vi "form_archive.vi"(0 "C7NI6703":T16, 1 "C2NI6071E 2":T10, 2 "C1NI6071E":T9, 3 "C6NI6703":T15, 5 "C1011NI6602":T14, 7 "C9NI6703":T11, 9 "C2NI6071E":T10, 12 "C5_IN_DIO96":T12, 13 "C8NI6703":T17, 14 "VAM-A":T13) -> (4 "archive out":T1)   [LabVIEW 2020]
uses:
  archive.ctl
  sync_type_def.ctl
  HT_type-def.ctl
  HF_type_def.ctl
  vacuum_type_def.ctl
  modulator_type_def.ctl
  water_cooling_type_def.ctl
  all_magnets_type_def.ctl
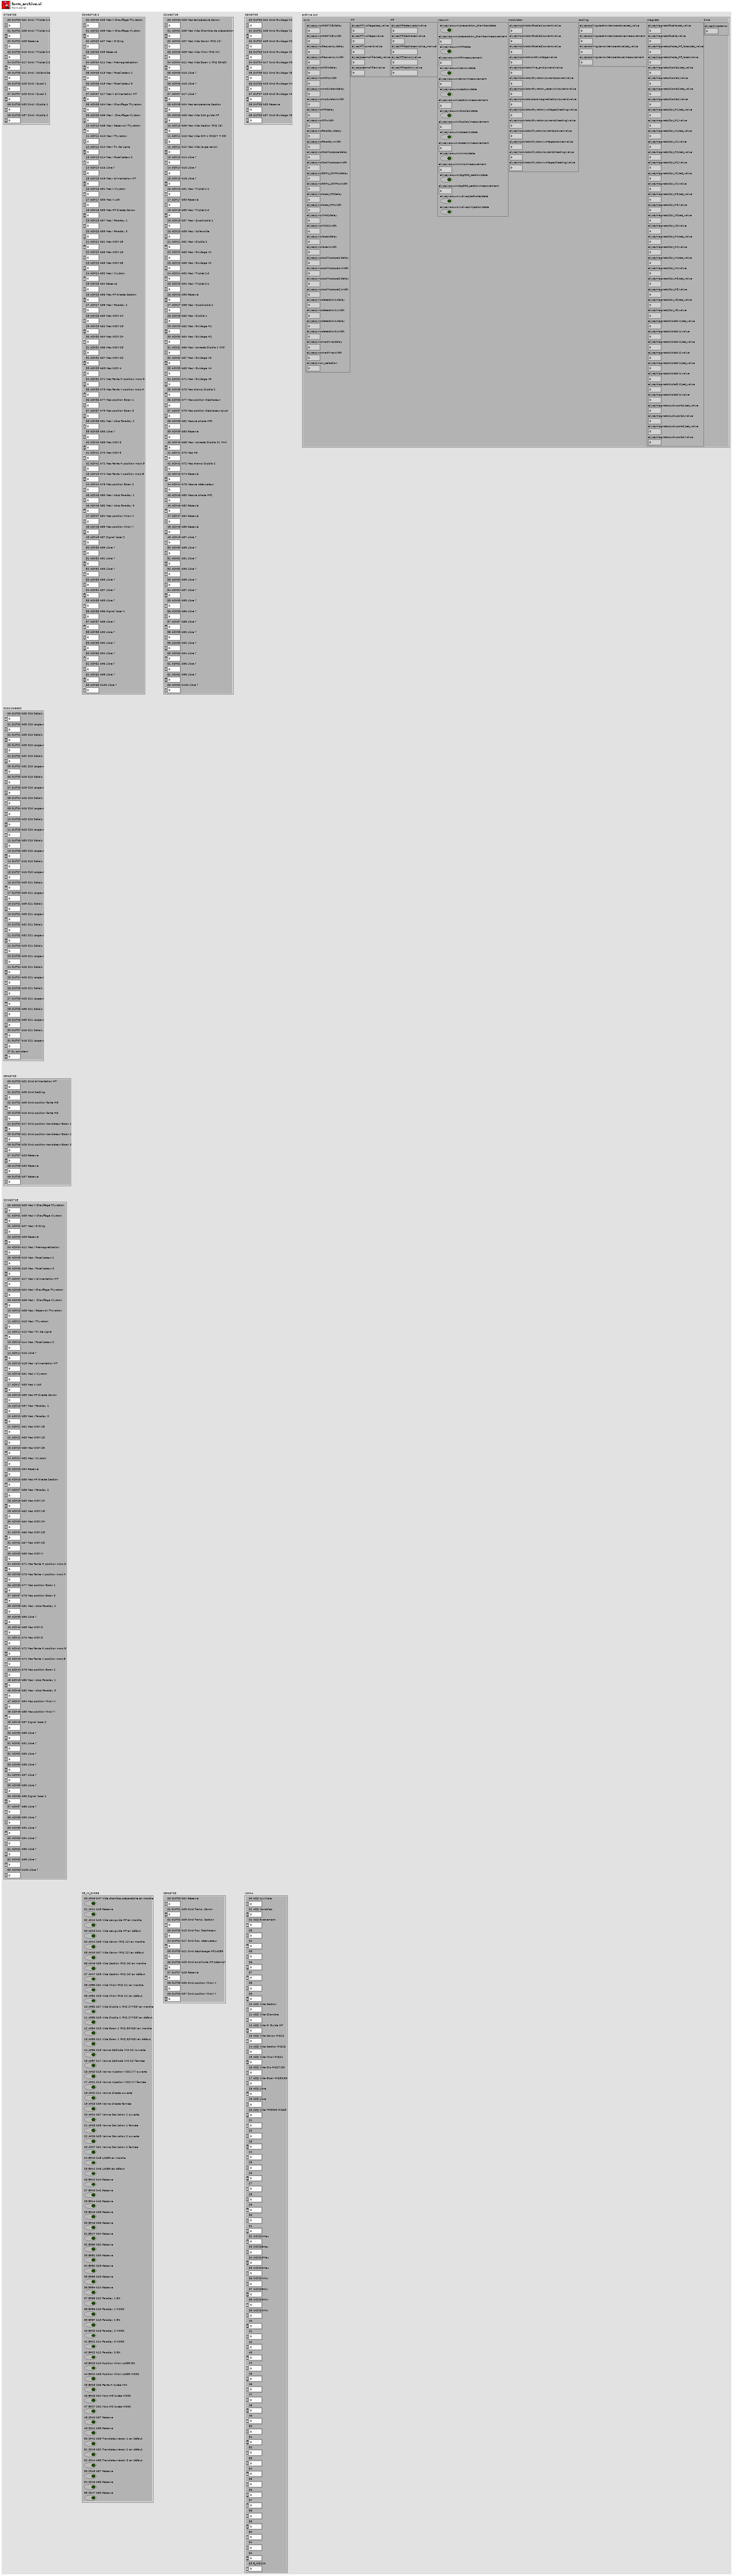
[diagram p1: front panel]
types:
  T1 = typedef "archive.ctl" = cluster{"sync":T2, "HT":T3, "HF":T4, "vacuum":T5, "modulator":T6, "cooling":T7, "magnets":T8, "time":cluster{"elyse/timestamp":dbl}}
  T2 = typedef "sync_type_def.ctl" = cluster{"elyse/sync/NI6071E/delay":dbl, "elyse/sync/NI6071E/width":dbl, "elyse/sync/frequency/delay":dbl, "elyse/sync/frequency/width":dbl, "elyse/sync/WCM/delay":dbl, "elyse/sync/WCM/width":dbl, "elyse/sync/modulator/delay":dbl, "elyse/sync/modulator/width":dbl, "elyse/sync/HF/delay":dbl, "elyse/sync/HF/width":dbl, "elyse/sync/Faraday/delay":dbl, "elyse/sync/Faraday/width":dbl, "elyse/sync/Oscilloscope/delay":dbl, "elyse/sync/Oscilloscope/width":dbl, "elyse/sync/50Hz_20MHz/delay":dbl, "elyse/sync/50Hz_20MHz/width":dbl, "elyse/sync/laser_HF/delay":dbl, "elyse/sync/laser_HF/width":dbl, "elyse/sync/IMAC/delay":dbl, "elyse/sync/IMAC/width":dbl, "elyse/sync/laser/delay":dbl, "elyse/sync/laser/width":dbl, "elyse/sync/oscilloscope1/delay":dbl, "elyse/sync/oscilloscope1/width":dbl, "elyse/sync/oscilloscope2/delay":dbl, "elyse/sync/oscilloscope2/width":dbl, "elyse/sync/detection1/delay":dbl, "elyse/sync/detection1/width":dbl, "elyse/sync/detection1/delay":dbl, "elyse/sync/detection2/width":dbl, "elyse/sync/machine/delay":dbl, "elyse/sync/machine/width":dbl, "elyse/sync/n_selection":dbl}
  T3 = typedef "HT_type-def.ctl" = cluster{"elyse/HT/voltage/set_value":dbl, "elyse/HT/voltage/value":dbl, "elyse/HT/current/value":dbl, "elyse/preamplifier/set_value":dbl, "elyse/preamplifier/value":dbl}
  T4 = typedef "HF_type_def.ctl" = cluster{"elyse/HF/attenuator/value":dbl, "elyse/HF/dephaser/value":dbl, "elyse/HF/dephaser/value_manuel":dbl, "elyse/HF/canon/value":dbl, "elyse/HF/section/value":dbl}
  T5 = typedef "vacuum_type_def.ctl" = cluster{"elyse/vacuum/preparation_chamber/state":bool, "elyse/vacuum/preparation_chamber/measurement":dbl, "elyse/vacuum/HF/state":bool, "elyse/vacuum/HF/measurement":dbl, "elyse/vacuum/canon/state":bool, "elyse/vacuum/canon/measurement":dbl, "elyse/vacuum/section/state":bool, "elyse/vacuum/section/measurement":dbl, "elyse/vacuum/dipole1/state":bool, "elyse/vacuum/dipole1/measurement":dbl, "elyse/vacuum/screen1/state":bool, "elyse/vacuum/screen1/measurement":dbl, "elyse/vacuum/mirror/state":bool, "elyse/vacuum/mirror/measurement":dbl, "elyse/vacuum/tpg300_section/state":bool, "elyse/vacuum/tpg300_section/measurement":dbl, "elyse/vacuum/valves/cathode/state":bool, "elyse/vacuum/valves/injection/state":bool}
  T6 = typedef "modulator_type_def.ctl" = cluster{"elyse/modulator/focale1/current/value":dbl, "elyse/modulator/focale2/current/value":dbl, "elyse/modulator/focale3/current/value":dbl, "elyse/modulator/LAR/voltage/value":dbl, "elyse/modulator/line_end/current/value":dbl, "elyse/modulator/thyratron/currents/power/value":dbl, "elyse/modulator/thyratron_reservoir/current/value":dbl, "elyse/modulator/paramagnetization/current/value":dbl, "elyse/modulator/thyratron/voltages/heating/value":dbl, "elyse/modulator/thyratron/currents/heating/value":dbl, "elyse/modulator/klystron/currents/power/value":dbl, "elyse/modulator/klystron/voltages/power/value":dbl, "elyse/modulator/klystron/currents/heating/value":dbl, "elyse/modulator/klystron/voltages/heating/value":dbl}
  T7 = typedef "water_cooling_type_def.ctl" = cluster{"elyse/cooling/section/temperature/set_value":dbl, "elyse/cooling/section/temperature/measurement":dbl, "elyse/cooling/canon/temperature/set_value":dbl, "elyse/cooling/canon/temperature/measurement":dbl}
  T8 = typedef "all_magnets_type_def.ctl" = cluster{"elyse/magnets/focale/set_value":dbl, "elyse/magnets/focale/value":dbl, "elyse/magnets/phase_HF_laser/set_value":dbl, "elyse/magnets/phase_HF_laser/value":dbl, "elyse/magnets/dipole1/set_value":dbl, "elyse/magnets/dipole1/value":dbl, "elyse/magnets/dipole2/set_value":dbl, "elyse/magnets/dipole2/value":dbl, "elyse/magnets/Cor_H1/set_value":dbl, "elyse/magnets/Cor_H1/value":dbl, "elyse/magnets/Cor_V1/set_value":dbl, "elyse/magnets/Cor_V1/value":dbl, "elyse/magnets/Cor_H2/set_value":dbl, "elyse/magnets/Cor_H2/value":dbl, "elyse/magnets/Cor_V2/set_value":dbl, "elyse/magnets/Cor_V2/value":dbl, "elyse/magnets/Cor_H3/set_value":dbl, "elyse/magnets/Cor_H3/value":dbl, "elyse/magnets/Cor_V3/set_value":dbl, "elyse/magnets/Cor_V3/value":dbl, "elyse/magnets/Cor_H4/set_value":dbl, "elyse/magnets/Cor_H4/value":dbl, "elyse/magnets/Cor_V4/set_value":dbl, "elyse/magnets/Cor_V4/value":dbl, "elyse/magnets/Cor_H5/set_value":dbl, "elyse/magnets/Cor_H5/value":dbl, "elyse/magnets/Cor_V5/set_value":dbl, "elyse/magnets/Cor_V5/value":dbl, "elyse/magnets/triplet1-1/set_value":dbl, "elyse/magnets/triplet1-1/value":dbl, "elyse/magnets/triplet1-2/set_value":dbl, "elyse/magnets/triplet1-2/value":dbl, "elyse/magnets/triplet2-1/set_value":dbl, "elyse/magnets/triplet2-1/value":dbl, "elyse/magnets/triplet2-2/set_value":dbl, "elyse/magnets/triplet2-2/value":dbl, "elyse/magnets/qudrupole1/set_value":dbl, "elyse/magnets/qudrupole1/value":dbl, "elyse/magnets/qudrupole2/set_value":dbl, "elyse/magnets/qudrupole2/value":dbl}
  T9 = cluster{"00 ACH00 b03 Mes température Canon":dbl, "01 ACH01 b05 Mes Vide Chambre de préparation":dbl, "02 ACH02 b07 Mes Vide Canon (PIQ 12)":dbl, "03 ACH03 b09 Mes Vide Miroir (PIQ 21)":dbl, "04 ACH04 b11 Mes Vide Ecran 1 (PIQ 53-63)":dbl, "05 ACH05 b13 Libre ?":dbl, "06 ACH06 b15 Libre ?":dbl, "07 ACH07 b17 Libre ?":dbl, "08 ACH08 b04 Mes température Section":dbl, "09 ACH09 b06 Mes Vide SAS guide HF":dbl, "10 ACH10 b08 Mes Vide Section (PIQ 16)":dbl, "11 ACH11 b10 Mes Vide DIP 1 (PIQ27 + 33)":dbl, "12 ACH12 b12 Mes Vide jauge canon":dbl, "13 ACH13 b14 Libre ?":dbl, "14 ACH14 b16 Libre ?":dbl, "15 ACH15 b18 Libre ?":dbl, "16 ACH16 b51 Mes I Triplet 1-1":dbl, "17 ACH17 b53 Réservé":dbl, "18 ACH18 b55 Mes I Triplet 2-2":dbl, "19 ACH19 b57 Mes I Quadripôle 1":dbl, "20 ACH20 b59 Mes I Solénoïde":dbl, "21 ACH21 b61 Mes I Dipôle 2":dbl, "22 ACH22 b63 Mes I Guidage V1":dbl, "23 ACH23 b65 Mes I Guidage V2":dbl, "24 ACH24 b52 Mes I Triplet 1-2":dbl, "25 ACH25 b54 Mes I Triplet 2-1":dbl, "26 ACH26 b56 Réservé":dbl, "27 ACH27 b58 Mes I Quadripôle 2":dbl, "28 ACH28 b60 Mes I Dipôle 1":dbl, "29 ACH29 b62 Mes I Guidage H1":dbl, "30 ACH30 b64 Mes I Guidage H2":dbl, "31 ACH31 b66 Mes I correcte Dipôle 1 (H3)":dbl, "32 ACH32 b67 Mes I Guidage V3":dbl, "33 ACH33 b69 Mes I Guidage V4":dbl, "34 ACH34 b71 Mes I Guidage V5":dbl, "35 ACH35 b73 Mes champ Dipôle 2":dbl, "36 ACH36 b77 Mes position Déphaseur":dbl, "37 ACH37 b79 Mes position Déphaseur ajust":dbl, "38 ACH38 b81 Mesure phase HF2":dbl, "39 ACH39 b83 Réservé":dbl, "40 ACH40 b68 Mes I correcte Dipôle 21 (H4)":dbl, "41 ACH41 b70 Mes H5":dbl, "42 ACH42 b72 Mes champ Dipôle 2":dbl, "43 ACH43 b74 Réservé":dbl, "44 ACH44 b78 Mesure Atténuateur":dbl, "45 ACH45 b80 Mesure phase HF1":dbl, "46 ACH46 b82 Réservé":dbl, "47 ACH47 b84 Réservé":dbl, "48 ACH48 b85 Réservé":dbl, "49 ACH49 b87 Libre ?":dbl, "50 ACH50 b89 Libre ?":dbl, "51 ACH51 b91 Libre ?":dbl, "52 ACH52 b93 Libre ?":dbl, "53 ACH53 b95 Libre ?":dbl, "54 ACH54 b97 Libre ?":dbl, "55 ACH55 b99 Libre ?":dbl, "56 ACH56 b86 Libre ?":dbl, "57 ACH57 b88 Libre ?":dbl, "58 ACH58 b90 Libre ?":dbl, "59 ACH59 b92 Libre ?":dbl, "60 ACH60 b94 Libre ?":dbl, "61 ACH61 b96 Libre ?":dbl, "62 ACH62 b98 Libre ?":dbl, "63 ACH63 b100 Libre ?":dbl}
  T10 = cluster{"00 ACH00 b03 Mes V Chauffage Thyratron":dbl, "01 ACH01 b05 Mes V Chauffage Klystron":dbl, "02 ACH02 b07 Mes I D'Qing":dbl, "03 ACH03 b09 Réservé":dbl, "04 ACH04 b11 Mes I Prémagnétisation":dbl, "05 ACH05 b13 Mes I Focalisateur 1":dbl, "06 ACH06 b15 Mes I Focalisateur 3":dbl, "07 ACH07 b17 Mes V alimentation HT":dbl, "08 ACH08 b04 Mes I Chauffage Thyratron":dbl, "09 ACH09 b06 Mes I  Chauffage Klystron":dbl, "10 ACH10 b08 Mes I Réservoir Thyratron":dbl, "11 ACH11 b10 Mes I Thyratron":dbl, "12 ACH12 b12 Mes I fin de Ligne":dbl, "13 ACH13 b14 Mes I Focalisateur 2":dbl, "14 ACH14 b16 Libre ?":dbl, "15 ACH15 b18 Mes I alimentation HT":dbl, "16 ACH16 b51 Mes V Klystron":dbl, "17 ACH17 b53 Mes V LAR":dbl, "18 ACH18 b55 Mes HF directe Canon":dbl, "19 ACH19 b57 Mes I Faraday 1":dbl, "20 ACH20 b59 Mes I Faraday 3":dbl, "21 ACH21 b61 Mes WCM 1B":dbl, "22 ACH22 b63 Mes WCM 1D":dbl, "23 ACH23 b65 Mes WCM 2B":dbl, "24 ACH24 b52 Mes I Klystron":dbl, "25 ACH25 b54 Réservé":dbl, "26 ACH26 b56 Mes HF directe Section":dbl, "27 ACH27 b58 Mes I Faraday 2":dbl, "28 ACH28 b60 Mes WCM 1H":dbl, "29 ACH29 b62 Mes WCM 1G":dbl, "30 ACH30 b64 Mes WCM 2H":dbl, "31 ACH31 b66 Mes WCM 2G":dbl, "32 ACH32 b67 Mes WCM 2D":dbl, "33 ACH33 b69 Mes WCM 4":dbl, "34 ACH34 b71 Mes Fente H position mors D":dbl, "35 ACH35 b73 Mes Fente V position mors H":dbl, "36 ACH36 b77 Mes position Ecran 1":dbl, "37 ACH37 b79 Mes position Ecran 3":dbl, "38 ACH38 b81 Mes I obcs Faraday 2":dbl, "39 ACH39 b83 Libre ?":dbl, "40 ACH40 b68 Mes WCM 3":dbl, "41 ACH41 b70 Mes WCM 5":dbl, "42 ACH42 b72 Mes Fente H position mors G":dbl, "43 ACH43 b74 Mes Fente V position mors B":dbl, "44 ACH44 b78 Mes position Ecran 2":dbl, "45 ACH45 b80 Mes I obcs Faraday 1":dbl, "46 ACH46 b82 Mes I obcs Faraday 3":dbl, "47 ACH47 b84 Mes position Miroir X":dbl, "48 ACH48 b85 Mes position Miroir Y":dbl, "49 ACH49 b87 Signal laser 2":dbl, "50 ACH50 b89 Libre ?":dbl, "51 ACH51 b91 Libre ?":dbl, "52 ACH52 b93 Libre ?":dbl, "53 ACH53 b95 Libre ?":dbl, "54 ACH54 b97 Libre ?":dbl, "55 ACH55 b99 Libre ?":dbl, "56 ACH56 b86 Signal laser 1":dbl, "57 ACH57 b88 Libre ?":dbl, "58 ACH58 b90 Libre ?":dbl, "59 ACH59 b92 Libre ?":dbl, "60 ACH60 b94 Libre ?":dbl, "61 ACH61 b96 Libre ?":dbl, "62 ACH62 b98 Libre ?":dbl, "63 ACH63 b100 Libre ?":dbl}
  T11 = cluster{"00 OUT00 b01 Cmd alimentation HT":dbl, "01 OUT01 b05 Cmd DeQing":dbl, "02 OUT02 b09 Cmd position fente HG":dbl, "03 OUT03 b13 Cmd position fente HD":dbl, "04 OUT04 b17 Cmd position translateur Ecran 1":dbl, "05 OUT05 b21 Cmd position translateur Ecran 2":dbl, "06 OUT06 b25 Cmd position translateur Ecran 3":dbl, "07 OUT07 b29 Réserve":dbl, "08 OUT08 b33 Réserve":dbl, "09 OUT09 b37 Réserve":dbl}
  T12 = cluster{"00 APA0 b47 Vide chambre préparatoire en marche":bool, "01 APA1 b45 Réserve":bool, "02 APA2 b43 Vide sas guide HF en marche":bool, "03 APA3 b41 Vide sas guide HF en défaut":bool, "04 APA4 b39 Vide Canon (PIQ 12) en marche":bool, "05 APA5 b37 Vide Canon (PIQ 12) en défaut":bool, "06 APA6 b35 Vide Section (PIQ 16) en marche":bool, "07 APA7 b33 Vide Section (PIQ 16) en défaut":bool, "08 APB0 b31 Vide Miroir (PIQ 21) en marche":bool, "09 APB1 b29 Vide Miroir (PIQ 21) en défaut":bool, "10 APB2 b27 Vide Dipôle 1 (PIQ 27+33) en marche":bool, "11 APB3 b25 Vide Dipôle 1 (PIQ 27+33) en défaut":bool, "12 APB4 b23 Vide Ecran 1 (PIQ 53+63) en marche":bool, "13 APB5 b21 Vide Ecran 1 (PIQ 53+63) en défaut":bool, "14 APB6 b19 Vanne Cathode (VIC 01) ouverte":bool, "15 APB7 b17 Vanne Cathode (VIC 01) fermée":bool, "16 APC0 b15 Vanne Injection (VSC 17) ouverte":bool, "17 APC1 b13 Vanne Injection (VSC 17) fermée":bool, "18 APC2 b11 Vanne directe ouverte":bool, "19 APC3 b09 Vanne directe fermée":bool, "20 APC4 b07 Vanne Déviation 1 ouverte":bool, "21 APC5 b05 Vanne Déviation 1 fermée":bool, "22 APC6 b03 Vanne Déviation 2 ouverte":bool, "23 APC7 b01 Vanne Déviation 2 fermée":bool, "24 BPA0 b48 LASER en marche":bool, "25 BPA1 b46 LASER eb défaut":bool, "26 BPA2 b44 Réserve":bool, "27 BPA3 b42 Réserve":bool, "28 BPA4 b40 Réserve":bool, "29 BPA5 b38 Réserve":bool, "30 BPA6 b36 Réserve":bool, "31 BPA7 b34 Réserve":bool, "32 BPB0 b32 Réserve":bool, "33 BPB1 b30 Réserve":bool, "34 BPB2 b28 Réserve":bool, "35 BPB3 b26 Réserve":bool, "36 BPB4 b24 Réserve":bool, "37 BPB5 b22 Faraday 1 EN":bool, "38 BPB6 b20 Faraday 1 HORS":bool, "39 BPB7 b18 Faraday 2 EN":bool, "40 BPC0 b16 Faraday 2 HORS":bool, "41 BPC1 b14 Faraday 3 HORS":bool, "42 BPC2 b12 Faraday 3 EN":bool, "43 BPC3 b10 Position Miroir LASER EN":bool, "44 BPC4 b08 Position Miroir LASER HORS":bool, "45 BPC5 b06 Fente H butée MIN":bool, "46 BPC6 b04 Mors HG butée HORS":bool, "47 BPC7 b02 Mors HD butée HORS":bool, "48 CPA0 b97 Réserve":bool, "49 CPA1 b95 Réserve":bool, "50 CPA2 b93 Translateur écran 1 en défaut":bool, "51 CPA3 b91 Translateur écran 2 en défaut":bool, "52 CPA4 b89 Translateur écran 3 en défaut":bool, "53 CPA5 b87 Réserve":bool, "54 CPA6 b85 Réserve":bool, "55 CPA7 b83 Réserve":bool}
  T13 = cluster{"00 ACQ Auxiliare":dbl, "01 ACQ Variables":dbl, "02 ACQ Evénement":dbl, "03 ":dbl, "04":dbl, "05":dbl, "06":dbl, "07":dbl, "08":dbl, "09":dbl, "10 ACQ Vide Section":dbl, "11 ACQ Vide Chambre":dbl, "12 ACQ Vide PI Guide HF":dbl, "13 ACQ Vide Canon PIQ12":dbl, "14 ACQ Vide Section PIQ16":dbl, "15 ACQ Vide Miroir PIQ21":dbl, "16 ACQ Vide Dip PIQ27/33 ":dbl, "17 ACQ Vide Ecran PIQ53/63":dbl, "18 ACQ Libre":dbl, "19 ACQ Libre":dbl, "20 ACQ Vide TPG300 PIQ63":dbl, "21":dbl, "22":dbl, "23":dbl, "24":dbl, "25":dbl, "26":dbl, "27":dbl, "28":dbl, "29":dbl, "30":dbl, "31":dbl, "32 WCM2HMax":dbl, "33 WCM2BMax":dbl, "34 WCM2GMax":dbl, "35 WCM2DMax":dbl, "36 WCM2HMin":dbl, "37 WCM2BMin":dbl, "38 WCM2GMin":dbl, "39 WCM2DMin":dbl, "40":dbl, "41":dbl, "42":dbl, "43":dbl, "44":dbl, "45":dbl, "46":dbl, "47":dbl, "48":dbl, "49":dbl, "50":dbl, "51":dbl, "52":dbl, "53":dbl, "54":dbl, "55":dbl, "56":dbl, "57":dbl, "58":dbl, "59":dbl, "60":dbl, "61":dbl, "62":dbl, "63 B_NI6220":dbl}
  T14 = cluster{"00 OUT00 b05 C10 Délais":dbl, "01 OUT00 b05 C10 Largeur":dbl, "02 OUT01 b09 C10 Délais":dbl, "03 OUT01 b09 C10 Largeur":dbl, "04 OUT02 b32 C10 Délais":dbl, "05 OUT02 b32 C10 Largeur":dbl, "06 OUT03 b29 C10 Délais":dbl, "07 OUT03 b29 C10 Largeur":dbl, "08 OUT04 b26 C10 Délais":dbl, "09 OUT04 b26 C10 Largeur":dbl, "10 OUT05 b23 C10 Délais":dbl, "11 OUT05 b23 C10 Largeur":dbl, "12 OUT06 b53 C10 Délais":dbl, "13 OUT06 b53 C10 Largeur":dbl, "14 OUT07 b16 C10 Délais":dbl, "15 OUT07 b16 C10 Largeur":dbl, "16 OUT00 b05 C11 Délais":dbl, "17 OUT00 b05 C11 Largeur":dbl, "18 OUT01 b09 C11 Délais":dbl, "19 OUT01 b09 C11 Largeur":dbl, "20 OUT02 b32 C11 Délais":dbl, "21 OUT02 b32 C11 Largeur":dbl, "22 OUT03 b29 C11 Délais":dbl, "23 OUT03 b29 C11 Largeur":dbl, "24 OUT04 b26 C11 Délais":dbl, "25 OUT04 b26 C11 Largeur":dbl, "26 OUT05 b23 C11 Délais":dbl, "27 OUT05 b23 C11 Largeur":dbl, "28 OUT06 b53 C11 Délais":dbl, "29 OUT06 b53 C11 Largeur":dbl, "30 OUT07 b16 C11 Délais":dbl, "31 OUT07 b16 C11 Largeur":dbl, "N° du compteur":dbl}
  T15 = cluster{"00 OUT00 b01 Cmd Guidage H1":dbl, "01 OUT01 b05 Cmd Guidage V1":dbl, "02 OUT02 b09 Cmd Guidage H2":dbl, "03 OUT03 b13 Cmd Guidage V2":dbl, "04 OUT04 b17 Cmd Guidage H3":dbl, "05 OUT05 b21 Cmd Guidage V3":dbl, "06 OUT06 b25 Cmd Guidage H4":dbl, "07 OUT07 b29 Cmd Guidage V4":dbl, "08 OUT08 b33 Réserve":dbl, "09 OUT09 b37 Cmd Guidage V5":dbl}
  T16 = cluster{"00 OUT00 b01 Cmd I Triplet 1-1":dbl, "01 OUT01 b05 Cmd I Triplet 1-2":dbl, "02 OUT02 b09 Réserve":dbl, "03 OUT03 b13 Cmd I Triplet 2-1":dbl, "04 OUT04 b17 Cmd I Triplet 2-2":dbl, "05 OUT05 b21 Cmd I Solénoïde":dbl, "06 OUT06 b25 Cmd I Quad 1":dbl, "07 OUT07 b29 Cmd I Quad 2":dbl, "08 OUT08 b33 Cmd I Dipôle 1":dbl, "09 OUT09 b37 Cmd I Dipôle 2":dbl}
  T17 = cluster{"00 OUT00 b01 Réserve":dbl, "01 OUT01 b05 Cmd Temp. Canon":dbl, "02 OUT02 b09 Cmd Temp. Section":dbl, "03 OUT03 b13 Cmd Pos. Déphaseur":dbl, "04 OUT04 b17 Cmd Pos. Atténuateur":dbl, "05 OUT05 b21 Cmd déphasage HF/LASER":dbl, "06 OUT06 b25 Cmd amplitude HF préampli":dbl, "07 OUT07 b29 Réserve":dbl, "08 OUT08 b33 Cmd position Miroir X":dbl, "09 OUT09 b37 Cmd position Miroir Y":dbl}
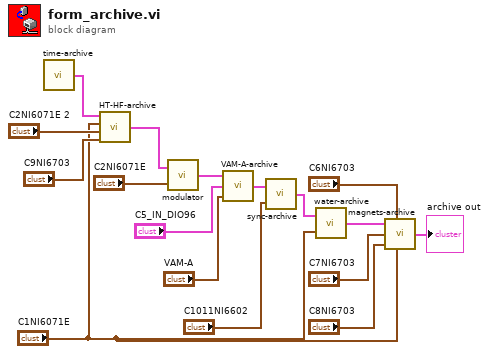
[diagram p0: block diagram]
diagram:
  n1 = call "time-archive.vi"() -> ("output cluster"=w5:T1)
  n2 = call "HT-HF-archive.vi"("C9NI6703"="C9NI6703", "C2NI6071E"="C2NI6071E 2", "C1NI6071E"="C1NI6071E", "archive in"=w5) -> ("archive out"=w6:T1)
  n3 = call "modulator.vi"("C2NI6071E"="C2NI6071E", "archive in"=w6) -> ("archive out"=w4:T1)
  n4 = call "VAM-A-archive.vi"("VAM-A"="VAM-A", "C5_IN_DIO96"="C5_IN_DIO96", "archive in"=w4) -> ("archive out"=w3:T1)
  n5 = call "sync-archive.vi"("C1011NI6602"="C1011NI6602", "archive in"=w3) -> ("archive out"=w2:T1)
  n6 = call "water-archive.vi"("C1NI6071E"="C1NI6071E", "archive in"=w2) -> ("archive out"=w1:T1)
  n7 = call "magnets-archive.vi"("archive in"=w1, "C6NI6703"="C6NI6703", "C7NI6703"="C7NI6703", "C8NI6703"="C8NI6703", "C1NI6071E"="C1NI6071E") -> ("archive out"=→"archive out":T1)
